vi "Write photo cal.vi"(6 "Photometer index":i32, 8 "error in (no error)":errorcluster, 9 "units":string, 11 "Photometer data in":T1) -> (0 "error out":errorcluster)   [LabVIEW 2019]
uses:
  Photometer calibration data.ctl
  DAQ configuration/Sensor buffer command.ctl
  DAQ configuration/scale type.ctl
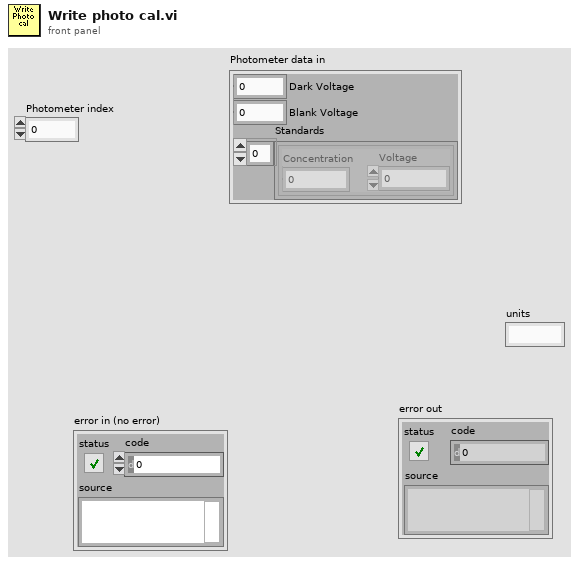
[diagram p1: front panel]
types:
  T1 = typedef "Photometer calibration data.ctl" = cluster{"Dark Voltage":dbl, "Blank Voltage":dbl, "Standards":cluster{"Concentration":dbl, "Voltage":dbl}[]}
  T2 = typedef "scale type.ctl" = enum16{"Volts", "Polynomial", "Correspondence Table", "pH", "Dissolved Oxygen", "Quadratic", "Photometer"}
  T3 = typedef "Sensor buffer command.ctl" = enum16{"read average", "read recent", "read all", "write", "set buffer size", "Read channel config", "Write channel config", "clear"}
  T4 = typedef "Channel config.ctl" = cluster{"Channel Indices":T5[], "AI Max voltage":dbl[], "Calibration matrix":T6}
  T5 = typedef "channel identifier.ctl" = u16
  T6 = typedef "calib array.ctl" = T7[]
  T7 = typedef "conversion.ctl" = cluster{"conversion matrix":sgl[][], "units":string, "name":string, "scale type":T2, "offset (volts)":dbl, "second channel":i8, "correspondence table":T8, "offset (physical units)":dbl, "pH scale":T9, "D.O.":T10, "Photometer data":T1}
  T8 = typedef "correspondence table.ctl" = cluster{"physical units":dbl, "volts":dbl}[]
  T9 = typedef "pH scale.ctl" = cluster{"Buffers":cluster{"Buffer":dbl, "Calibrated":bool, "V/T":dbl}[], "Temperature":dbl}
  T10 = typedef "DO scale.ctl" = cluster{"Temperature":dbl, "K":dbl, "barometric pressure":dbl}
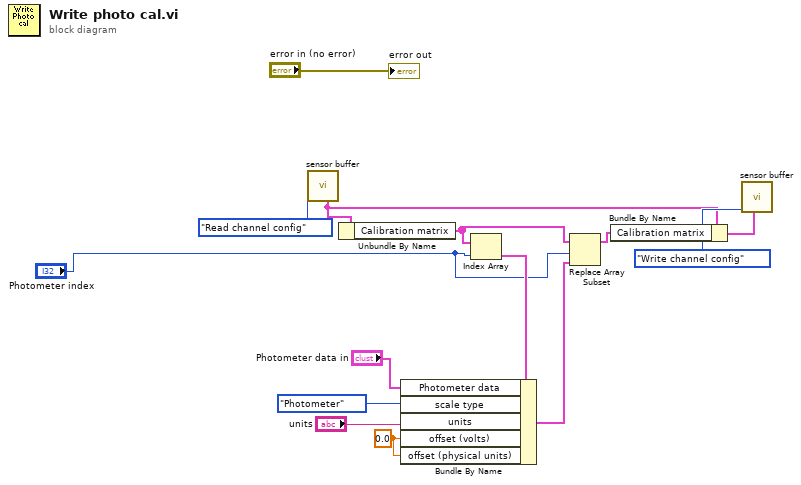
[diagram p0: block diagram]
diagram:
  w1 = 0.0 ("offset (volts)")
  n1 = call "sensor buffer.vi"("command"=Sensor_buffer_command."Read channel config") -> ("Channel Config out"=w12:T4)  [unwired: 6 in, 4 out]
  n2 = Unbundle By Name(w12) -> ("Calibration matrix"=w8:T6)
  n3 = Index Array(array=w8, index="Photometer index") -> (element=w10:T7)
  n4 = Bundle By Name(cluster=w10, "Photometer data"="Photometer data in", "scale type"=scale_type."Photometer", "units"="units", "offset (volts)"=w1, "offset (physical units)"=w1) -> (w9:T7)
  n5 = Replace Array Subset(array=w8, new element=w9, index="Photometer index") -> (w7:T6)
  n6 = Bundle By Name(cluster=w12, "Calibration matrix"=w7) -> (w11:T4)
  n7 = call "sensor buffer.vi"("Channel Config"=w11, "command"=Sensor_buffer_command."Write channel config") -> ()  [unwired: 5 in, 5 out]
  "error out" <- "error in (no error)"
